vi "Obtian Read Queue.vi"(7 "ID":i32, 8 "error in (no error)":errorcluster, 10 "Read Queue Array":T1[](array[typedef]), 11 "CAN Session Queue":T2) -> (0 "error out":errorcluster, 3 "ID Read Queue":refnum<queue>)   [LabVIEW 2016]
uses:
  Program Files (x86)/National Instruments/LabVIEW 2016/examples/robotics/EPOS2 CANOpen Driver/Low Level VIs/Typedefs/CAN Session Pointer.ctl
  Program Files (x86)/National Instruments/LabVIEW 2016/examples/robotics/EPOS2 CANOpen Driver/Low Level VIs/Typedefs/CAN Communication References.ctl
  Program Files (x86)/National Instruments/LabVIEW 2016/examples/robotics/EPOS2 CANOpen Driver/Low Level VIs/Typedefs/kill process notifier array.ctl
  Program Files (x86)/National Instruments/LabVIEW 2016/examples/robotics/EPOS2 CANOpen Driver/Low Level VIs/Typedefs/Write Queue.ctl
  Program Files (x86)/National Instruments/LabVIEW 2016/examples/robotics/EPOS2 CANOpen Driver/Low Level VIs/Typedefs/FPGA CAN Frame Cluster.ctl
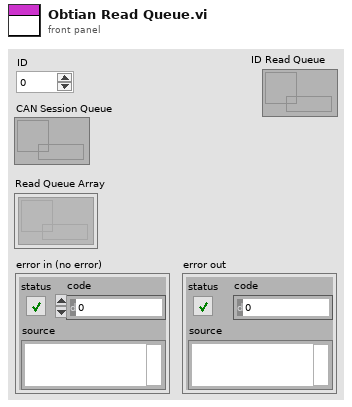
[diagram p1: front panel]
types:
  T1 = typedef "Write Queue.ctl" = refnum<queue>
  T2 = typedef "CAN Session Pointer.ctl" = refnum<queue>
  T3 = cluster{"Timestamp":u64, "Identifier":u32, "Type":u8, "InfoA":u8, "InfoB":u8, "DataLength":u8, "Data":u8[]}
  T4 = typedef "CAN Communication References.ctl" = cluster{"kill process notifier array":T5, "Write Queue":T1, "New Frame Notifier":refnum<notifier>, "Read Queue Array":T1[]}
  T5 = typedef "kill process notifier array.ctl" = refnum<notifier>[]
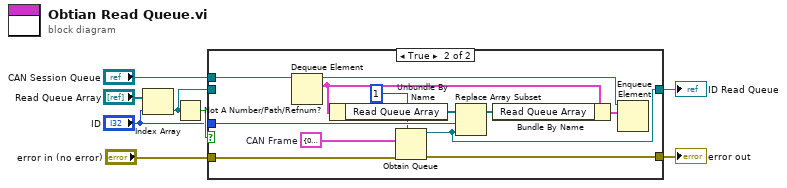
[diagram p0: block diagram]
diagram:
  n1 = Index Array(array="Read Queue Array", index="ID") -> (element=w3:T1)
  n2 = Not A Number/Path/Refnum?(number/path/refnum=w3) -> (NaN/Path/Refnum?=w8:bool)
  n3 = case shown="True" w8 {
    tunnel: "ID" -> [_ w22]
    tunnel: "CAN Session Queue" -> [_ w20]
    tunnel: [w10 w14] -> w4
    tunnel: w3 -> [w10 _]
    tunnel: "error in (no error)" -> [w9 w13]
    tunnel: [w9 w12] -> w1
    frame False {
    }
    frame True {
      w21 = T3 {"Timestamp"=0, "Identifier"=0, "Type"=0, "InfoA"=0, "InfoB"=0, "DataLength"=0, "Data"=[0, 0, 0, 0, 0, 0, 0, 0]}  # CAN Frame
      n4 = Dequeue Element(queue=w20) -> (queue out=w15:T2, element=w18:T4)  [unwired: 2 in, 2 out]
      n5 = Unbundle By Name(w18) -> ("Read Queue Array"=w19:T1[])
      n6 = Obtain Queue(max queue size (-1, unlimited)=1, element data type=w21, error in (no error)=w13) -> (queue out=w14:refnum<queue>, error out=w12:errorcluster)  [unwired: 2 in, 1 out]
      n7 = Replace Array Subset(array=w19, new element=w14, index=w22) -> (w17:T1[])
      n8 = Bundle By Name(cluster=w18, "Read Queue Array"=w17) -> (w16:T4)
      n9 = Enqueue Element(queue=w15, element=w16) -> ()  [unwired: 2 in, 3 out]
    }
  }
  "ID Read Queue" <- w4
  "error out" <- w1
